vi "Get Sheet Number.vi"(8 "error in (no error)":errorcluster, 11 "Document in":refnum<class "Document.lvclass">) -> (0 "error out":errorcluster, 2 "Excel.Workbook.Sheet Number":i32, 3 "Document out":refnum<class "Document.lvclass">)   [LabVIEW 2017, in "LabVIEW NPOI.lvlib" / "Document.lvclass"]
uses:
  Document.lvclass
  MS-Excel/MS-Excel.lvclass
  <vilib>/Utility/error.llb/Error Cluster From Error Code.vi
  <vilib>/ErrorRing/Error Ring.xnode
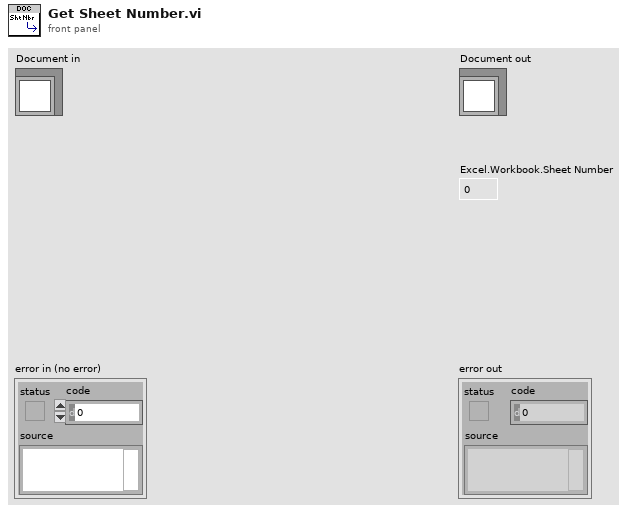
[diagram p1: front panel]
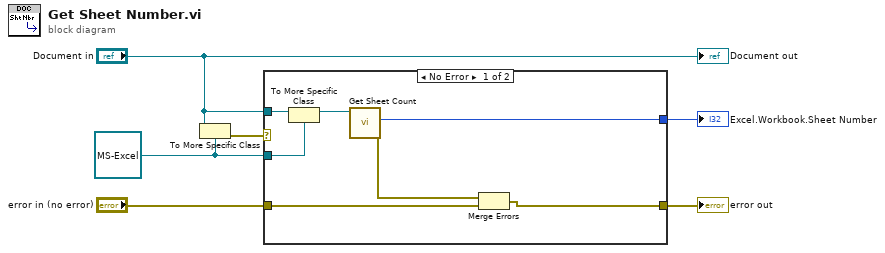
[diagram p0: block diagram]
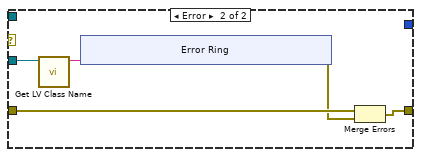
[diagram p2: hidden frame]
diagram:
  w5 = refnum<class "MS-Excel.lvclass"> refnum ("LabVIEW NPOI.lvlib:MS-Excel.lvclass")
  n1 = To More Specific Class(target class=w5, reference="Document in") -> (error out=w6:errorcluster)  [unwired: 1 in, 1 out]
  n2 = case shown="No Error" w6 {
    tunnel: "Document in" -> [w13 _]
    tunnel: w5 -> [w12 w18]
    tunnel: [w8 _] -> w1
    tunnel: "error in (no error)" -> [w10 w16]
    tunnel: [w11 w15] -> w2
    frame No Error {
      n3 = To More Specific Class(target class=w12, reference=w13) -> (specific class reference=w9:refnum<class "MS-Excel.lvclass">)  [unwired: 1 in, 1 out]
      n4 = call "Get Sheet Count.vi"("MS-Excel in"=w9) -> ("error out"=w7:errorcluster, "#Sheets"=w8:i32)  [unwired: 8 in, 1 out]
      n5 = Merge Errors(w7, w10) -> (w11:errorcluster)
    }
    frame Error {
      n6 = call <vilib>:"Get LV Class Name.vi"("object"=w18) -> ("class name"=w17:string)  [unwired: 9 in, 1 out]
      n7 = xnode "Error Ring"("parameter 0"=w17) -> ("error out"=w14:errorcluster)
      n8 = Merge Errors(w16, w14) -> (w15:errorcluster)
    }
  }
  "error out" <- w2
  "Excel.Workbook.Sheet Number" <- w1
  "Document out" <- "Document in"
